vi "Find Report Implementations.vi"(8 "error in (no error)":errorcluster, 11 "Report Generator In":refnum<class "Report Generator.lvclass">) -> (0 "error out":errorcluster, 1 "Active index":i32, 2 "Test Reports":string[](array[string]), 3 "Report Generator Out":refnum<class "Report Generator.lvclass">)   [LabVIEW 2020, in "Report Generator.lvclass"]
uses:
  Report Generator.lvclass
  Report Generator.lvclass/Report Generator.ctl
  Report Classes/Test Report/Test Report.lvclass
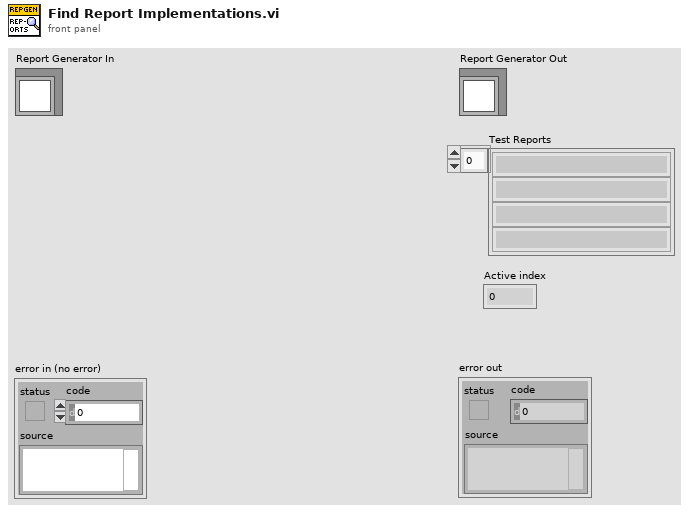
[diagram p1: front panel]
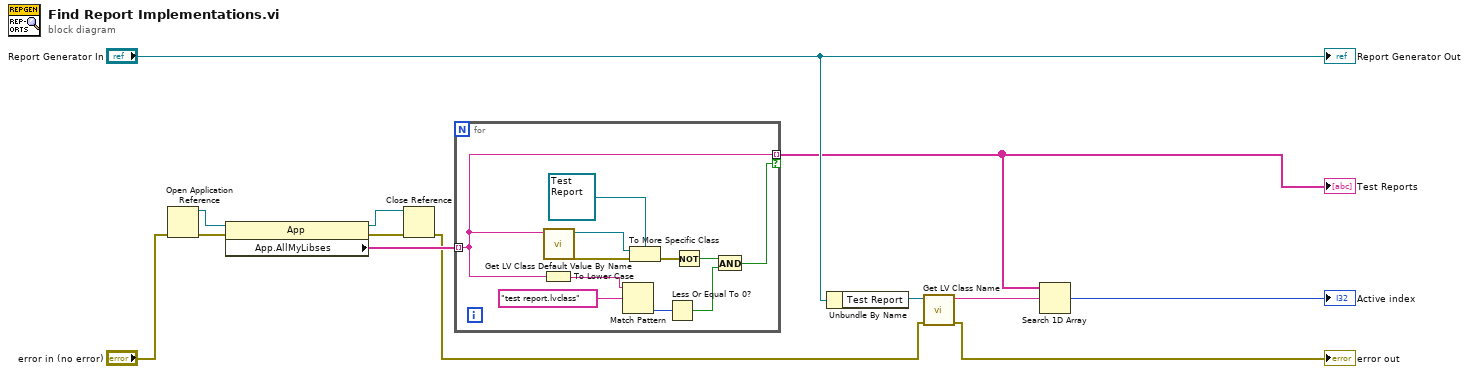
[diagram p0: block diagram]
diagram:
  n1 = Open Application Reference(8:"error in (no error)") -> (0:w12:errorcluster, 3:w13:refnum<vi>)  [unwired: 3 in]
  n2 = property class="App"(reference=w13, error in=w12) -> (reference out=w10:refnum<vi>, error out=w11:errorcluster, "App.AllMyLibses"=w9:string[])
  n3 = Close Reference(reference=w10, error in (no error)=w11) -> (error out=w3:errorcluster)
  n4 = for {
    tunnel: w9 -> [w18] mode=indexing
    tunnel: [w18] -> w1 mode=indexing if=w15
    n5 = To Lower Case(string=w18) -> (all lower case string=w16:string)
    n6 = call <vilib>:"Get LV Class Default Value By Name.vi"("class name"=w18) -> ("error out"=w24:errorcluster, "object"=w23:refnum<class>)  [unwired: 9 in]
    n7 = Match Pattern(string=w16, regular expression="test report.lvclass") -> (offset past match=w20:i32)  [unwired: 1 in, 3 out]
    n8 = To More Specific Class(target class=refnum<class "Test Report.lvclass"> refnum ("Test Report.lvclass"), reference=w23, error in=w24) -> (error out=w21:errorcluster)  [unwired: 1 out]
    n9 = Less Or Equal To 0?(x=w20) -> (x <= 0?=w14:bool)
    n10 = Not(x=w21) -> (.not. x?=w17:bool)
    n11 = And(x=w17, y=w14) -> (x .and. y?=w15:bool)
  }
  "Test Reports" <- w1
  n12 = Unbundle By Name("Report Generator In") -> ("Test Report"=w6:refnum<class "Test Report.lvclass">)
  n13 = call <vilib>:"Get LV Class Name.vi"("error in (no error)"=w3, "object"=w6) -> ("error out"=→"error out":errorcluster, "class name"=w5:string)  [unwired: 8 in]
  n14 = Search 1D Array(1D array=w1, element=w5) -> (index of element=→"Active index":i32)  [unwired: 1 in]
  "Report Generator Out" <- "Report Generator In"
